vi "Display.vi"(8 "error in":errorcluster, 11 "SVG Parent in":refnum<class "SVG Parent.lvclass">) -> (0 "error out":errorcluster, 3 "SVG Parent out":refnum<class "SVG Parent.lvclass">)   [LabVIEW 2019, in "Pop-Up.lvlib" / "SVG Parent.lvclass"]
doc: "This is the override method required for each child of the pop up class. It is the pop up that will display to the user.\n\nTo extend this function, create a child class of the pop up class. Then create an override method for this VI. <b>Display.vi</b> is a protected function, therefore it cannot be called in a main application. This VI must be called by a caller function. See one of the standard pop-ups for a setup example.\n\n<b>Code Developed By:</b>\nDaniel Coons\nTechnology Service Corporation\n1983 S Liberty Drive\nBloomington, IN 47403\nPhone: 812 558-7100\ndaniel.coons@tsc.com\nwww.tsc.com/atcs"
uses:
  SVG Parent.lvclass
  Popup/Popup.lvclass
panel:
  # "This VI displays the popup"
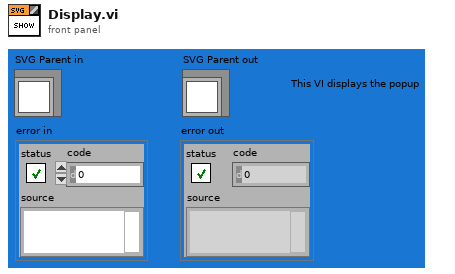
[diagram p1: front panel]
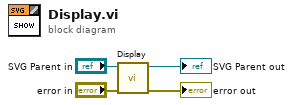
[diagram p0: block diagram]
diagram:
  n1 = call-parent "Display.vi"("error in"="error in", "Popup in"="SVG Parent in") -> ("error out"=→"error out":errorcluster, "Popup out"=→"SVG Parent out":refnum<class "SVG Parent.lvclass">)  [unwired: 8 in]
